vi "fm-demodulator.vi"() -> ()   [LabVIEW 2021]
panel:
  out "Segnale demodulato":dbl[](graph)
  out "Segnale FM":dbl[](graph)
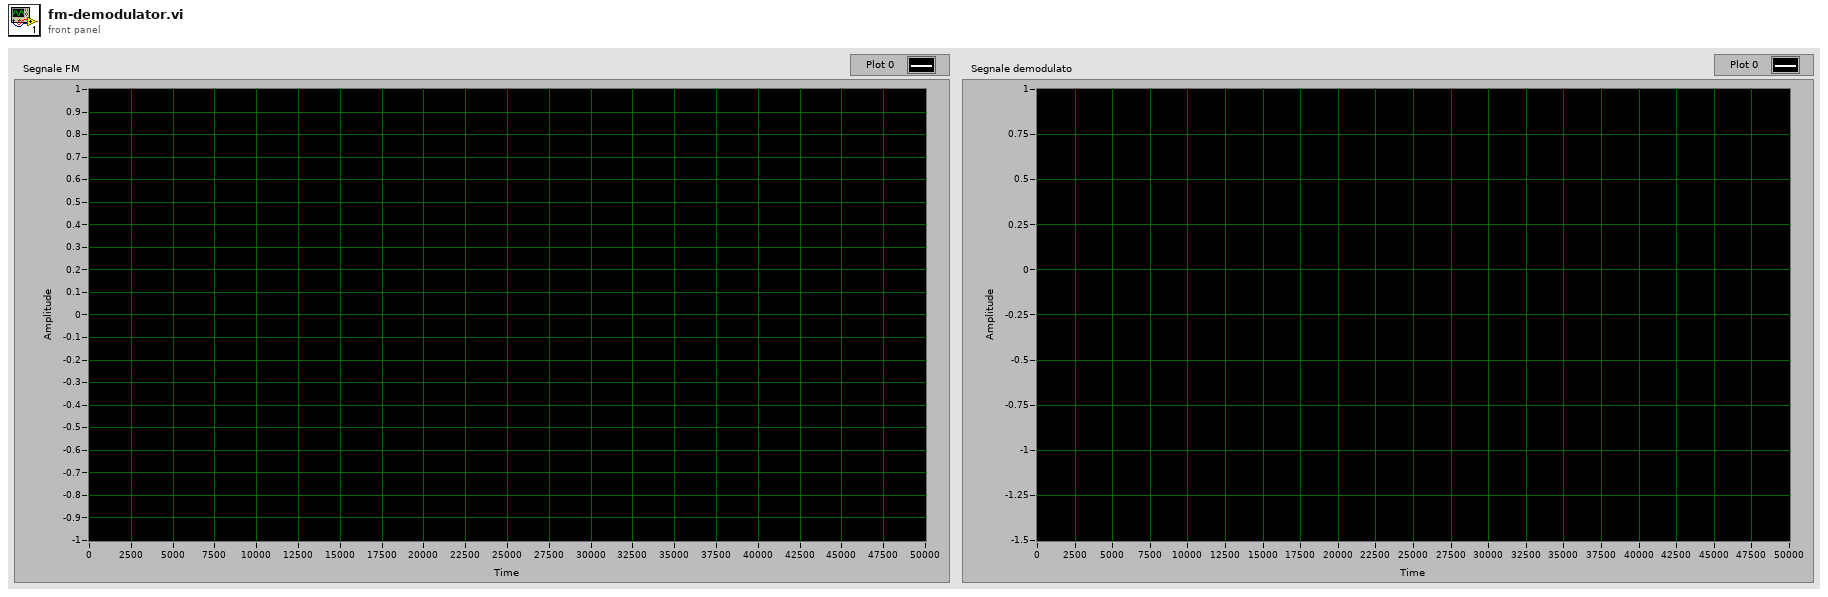
[diagram p1: front panel]
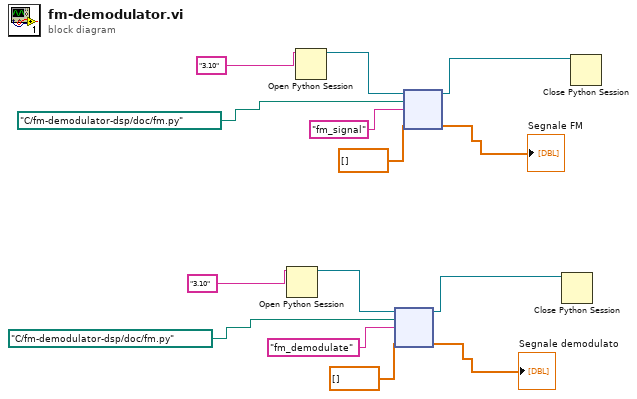
[diagram p0: block diagram]
diagram:
  n1 = Open Python Session(python version="3.10" ("Python version")) -> (session out=w7:refnum<k35>)  [unwired: 2 in, 1 out]
  n2 = Open Python Session(python version="3.10" ("Python version")) -> (session out=w14:refnum<k35>)  [unwired: 2 in, 1 out]
  n3 = node(w7, path "C:/fm-demodulator-dsp/doc/fm.py" ("name or relative path"), "fm_demodulate" ("function name"), dbl[] []) -> (w4:refnum<k35>, →"Segnale demodulato":dbl[])  [unwired: 1 in, 3 out]
  n4 = node(w14, path "C:/fm-demodulator-dsp/doc/fm.py" ("name or relative path"), "fm_signal" ("function name"), dbl[] []) -> (w11:refnum<k35>, →"Segnale FM":dbl[])  [unwired: 1 in, 3 out]
  n5 = Close Python Session(session in=w4) -> ()  [unwired: 1 in, 1 out]
  n6 = Close Python Session(session in=w11) -> ()  [unwired: 1 in, 1 out]
